vi "build_en_face_sequential.vi"(0 "Existing En Face":T1, 1 "Image to add":T1, 2 "current x":dbl, 3 "current y":dbl, 4 "depth":dbl, 5 "error in (no error)":errorcluster, 6 "aspect ratio":dbl, 7 "output line":i32, 9 "Track Surface":bool) -> (14 "En Face Image Out":T1)   [LabVIEW 2016]
uses:
  <vilib>/vision/Image Controls.llb/IMAQ Image.ctl
panel:
  out "Waveform Chart":dbl(graph)
  out "error out":errorcluster
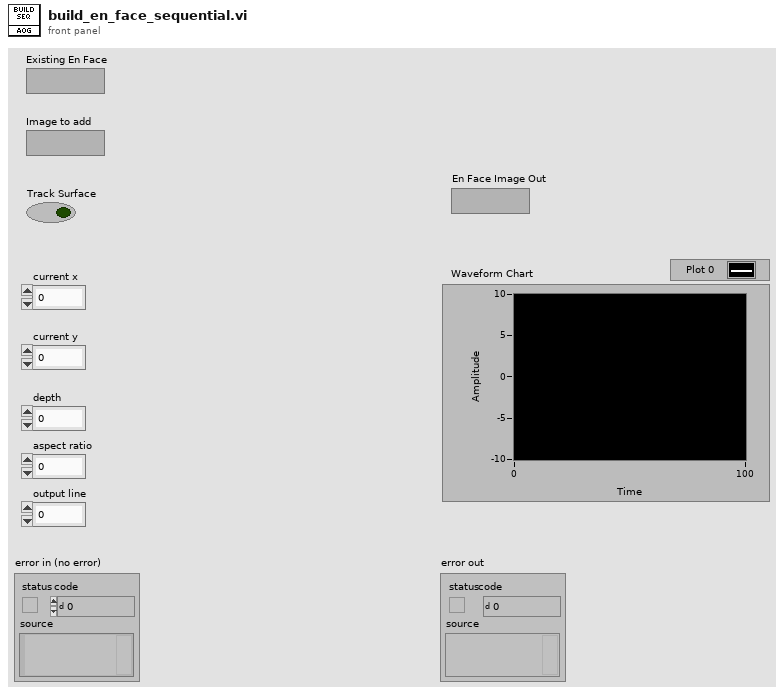
[diagram p1: front panel]
types:
  T1 = typedef "IMAQ Image.ctl" = refnum<image>
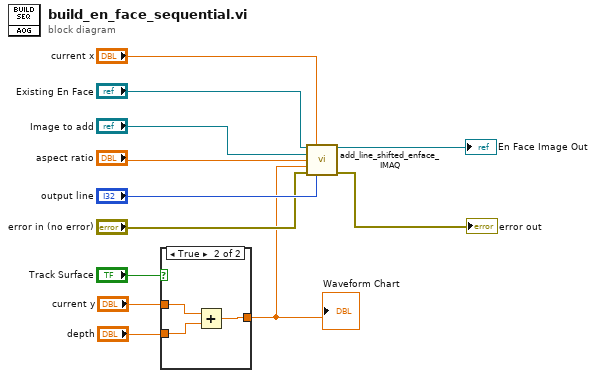
[diagram p0: block diagram]
diagram:
  n1 = case shown="True" "Track Surface" {
    tunnel: "depth" -> [w13 w16]
    tunnel: "current y" -> [_ w15]
    tunnel: [w13 w14] -> w1
    frame False {
    }
    frame True {
      n2 = Add(x=w15, y=w16) -> (x+y=w14:dbl)
    }
  }
  "Waveform Chart" <- w1
  n3 = call "add_line_shifted_enface_IMAQ.vi"("En Face Image"="Existing En Face", "Shift"="current x", "Raw Image"="Image to add", "Aspect Ratio"="aspect ratio", "Input Line"=w1, "error in (no error)"="error in (no error)", "Output Line"="output line") -> ("En Face Image Out"=→"En Face Image Out":T1, "error out"=→"error out":errorcluster)  [unwired: 7 in]
